vi "操作日志.vi"(8 "error in (no error)":errorcluster, 10 "table":string="操作日志", 11 "日志信息":string) -> (0 "error out":errorcluster)   [LabVIEW 2016, in "斯坦道多参数.lvlib"]
uses:
  <vilib>/addons/database/Auxilliary.llb/DB Tools Transaction.ctl
  <vilib>/addons/database/Auxilliary.llb/DB Tools Isolation Level.ctl
  <vilib>/Utility/sysdir.llb/System Directory Type.ctl
  <vilib>/addons/database/Connection.llb/DB Tools Open Connec (String).vi
  <vilib>/addons/database/Connection.llb/Conn Transaction.vi
  <vilib>/addons/database/NI_Database_API.lvlib
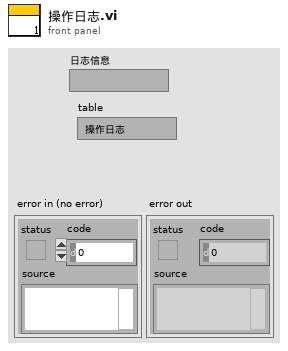
[diagram p1: front panel]
types:
  T1 = typedef "System Directory Type.ctl" = i32
  T2 = typedef "NI_Database_API.lvlib/DB Tools Isolation Level.ctl" = enum16{"chaos", "read uncommitted", "read committed", "repeatable read", "serializable"}
  T3 = typedef "NI_Database_API.lvlib/DB Tools Transaction.ctl" = enum16{"begin", "commit", "rollback"}
  T4 = cluster{"时间标识":timestamp, "设备":string, "日志信息":string, "流程参数":string}
  T5 = typedef "NI_Database_API.lvlib/Conn ObjectReference.ctl" = refnum<k1>
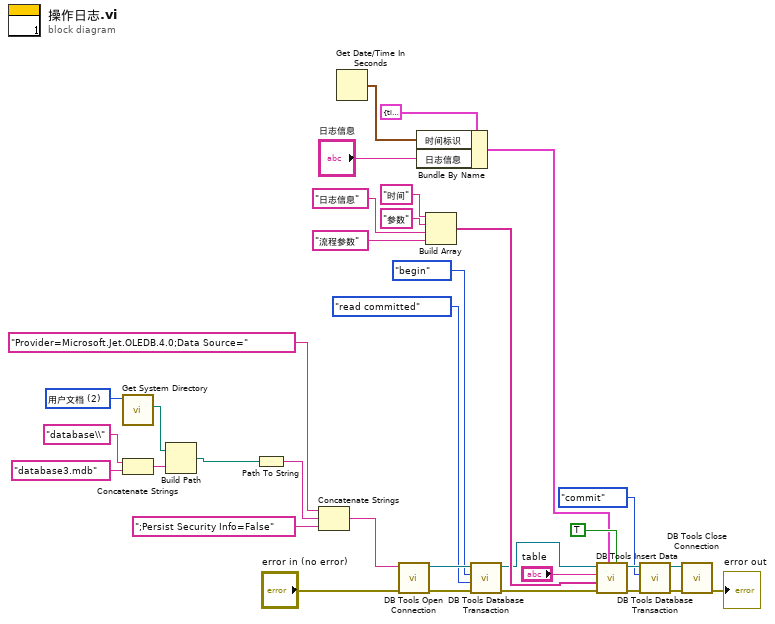
[diagram p0: block diagram]
diagram:
  w1 = T1 2 items=["用户目录"=0, "用户桌面"=1, "用户文档"=2, "用户应用程序数据"=3, "用户设置"=4, "用户临时目录"=5, "公共文档"=6, "公共应用程序数据"=7, "公共设置"=8, "公共缓存"=13, "系统核心库"=9, "系统安装库"=10, "应用程序文件"=11, "启动盘根目录"=12] ("system directory type")
  n1 = call <vilib>:"Get System Directory.vi"("system directory type"=w1) -> ("system directory"=w2:path)  [unwired: 10 in]
  n2 = Concatenate Strings("database\\" ("condition"), "database3.mdb" ("database")) -> (w4:string)
  n3 = Build Path(base path=w2, name or relative path=w4) -> (appended path=w8:path)
  n4 = Path To String(path=w8) -> (string=w28:string)
  n5 = Concatenate Strings("Provider=Microsoft.Jet.OLEDB.4.0;Data Source=" ("condition"), w28, ";Persist Security Info=False" ("condition")) -> (w26:string)
  n6 = Get Date/Time In Seconds() -> (seconds since 1Jan1904=w21:timestamp)
  n7 = call-poly <vilib>:"DB Tools Open Connection.vi"("error in (no error)"="error in (no error)", "connection information"=w26) -> ("error out"=w17:errorcluster, "connection reference"=w25:T5)  [unwired: 6 in]
  n8 = Bundle By Name(cluster=T4 {"时间标识"=timestamp(0 s since 1904-01-01), "设备"="多参数", "日志信息"="", "流程参数"=""} ("data in"), "时间标识"=w21, "日志信息"="日志信息") -> (w20:T4)
  n9 = Build Array("时间", "参数" ("元素"), "日志信息", "流程参数") -> (w23:string[])
  n10 = call-poly <vilib>:"DB Tools Database Transaction.vi"("error in (no error)"=w17, "isolation level (chaos)"=DB_Tools_Isolation_Level."read committed", "operation (begin)"=DB_Tools_Transaction."begin", "connection reference"=w25) -> ("error out"=w16:errorcluster, "connection reference out"=w18:T5)  [unwired: 2 in]
  n11 = call <vilib>:"DB Tools Insert Data.vi"("create table? (F)"=TRUE, "data"=w20, "error in (no error)"=w16, "columns"=w23, "table"="table", "connection reference"=w18) -> ("error out"=w13:errorcluster, "connection reference out"=w15:T5)  [unwired: 4 in]
  n12 = call-poly <vilib>:"DB Tools Database Transaction.vi"("error in (no error)"=w13, "operation (begin)"=DB_Tools_Transaction."commit", "connection reference"=w15) -> ("error out"=w12:errorcluster, "connection reference out"=w14:T5)  [unwired: 3 in]
  n13 = call <vilib>:"DB Tools Close Connection.vi"("error in (no error)"=w12, "connection reference"=w14) -> ("error out"=→"error out":errorcluster)  [unwired: 5 in]
